vi "RunFormAbort.vi"(8 "エラー入力（エラーなし）":errorcluster, 11 "配列":refnum<vi>[](array[refnum])) -> (0 "エラー出力":errorcluster)   [LabVIEW 2014]
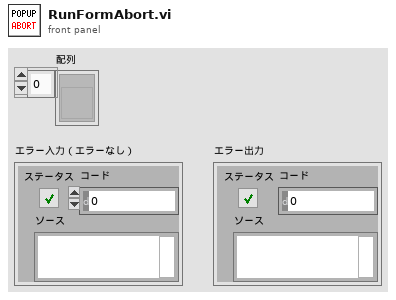
[diagram p1: front panel]
types:
  T1 = enum32{"Bad", "Idle", "Run top level", "Running"}
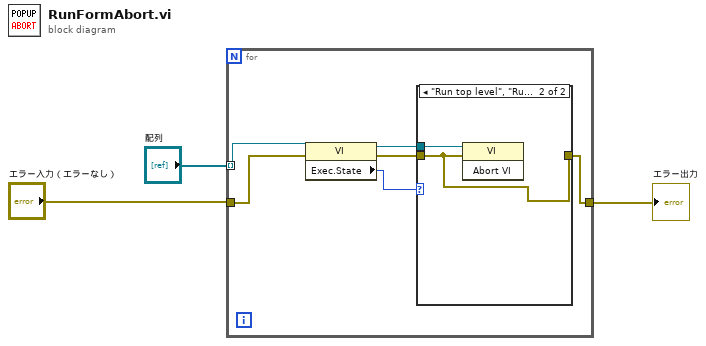
[diagram p0: block diagram]
diagram:
  n1 = for {
    tunnel: "配列" -> [w4] mode=indexing
    tunnel: "エラー入力（エラーなし）" -> [w6]
    tunnel: [w7] -> w1
    n2 = property class="VI"(reference=w4, error in=w6) -> (reference out=w9:refnum<vi>, error out=w5:errorcluster, "Exec.State"=w8:T1)
    n3 = case shown="\"Run top level\", \"Running\"" w8 {
      tunnel: w5 -> [w10 w11]
      tunnel: w9 -> [_ w12]
      tunnel: [w10 w11] -> w7
      frame "Bad", Default {
      }
      frame "Run top level", "Running" {
        n4 = invoke class="VI" method="Abort VI"(reference=w12, error in=w11) -> ()  [unwired: 1 in, 3 out]
      }
    }
  }
  "エラー出力" <- w1
